vi "Joystickdrivemotor.vi"(6 "Max Output":dbl=1.0, 7 "Square Inputs":bool=TRUE, 8 "right y":dbl, 9 "Y axis value":dbl, 10 "X axis value":dbl) -> (0 "Boolean 2":bool, 1 "Right Motor Value":dbl, 2 "Left Motor Value":dbl)   [LabVIEW 2015]
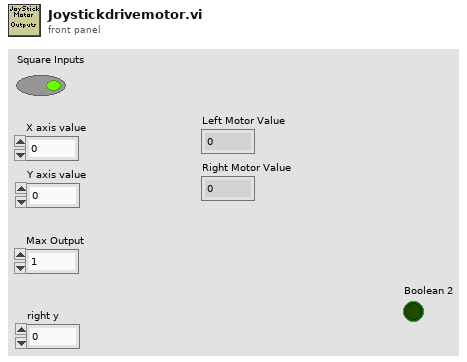
[diagram p1: front panel]
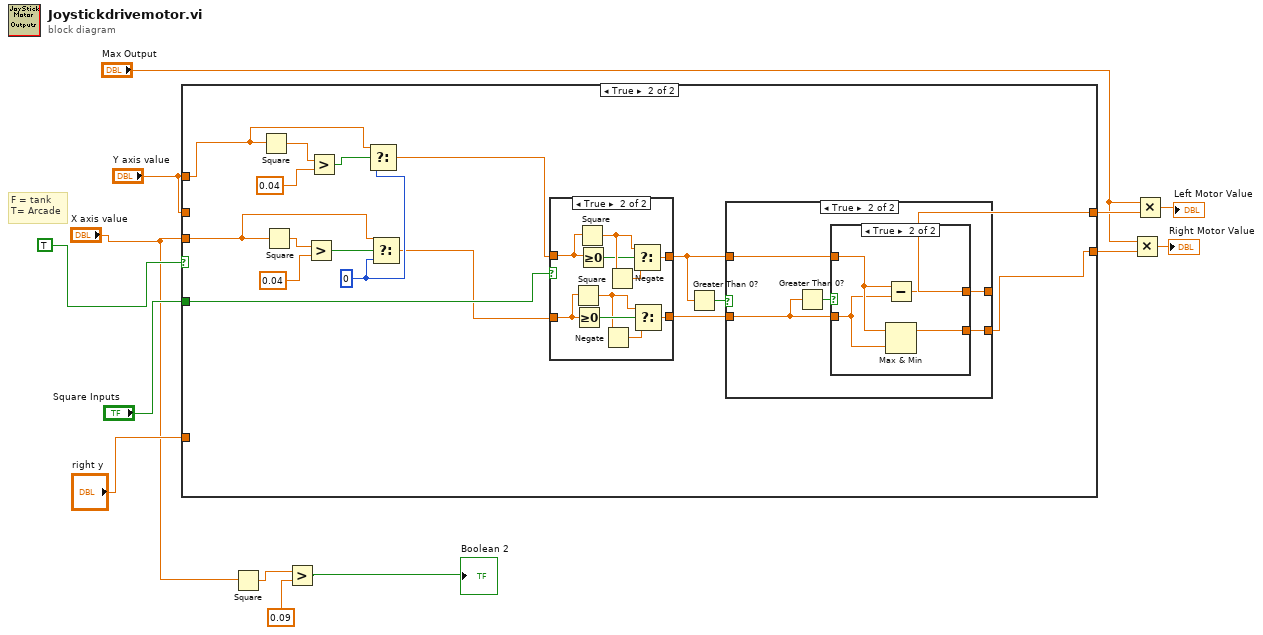
[diagram p0: block diagram]
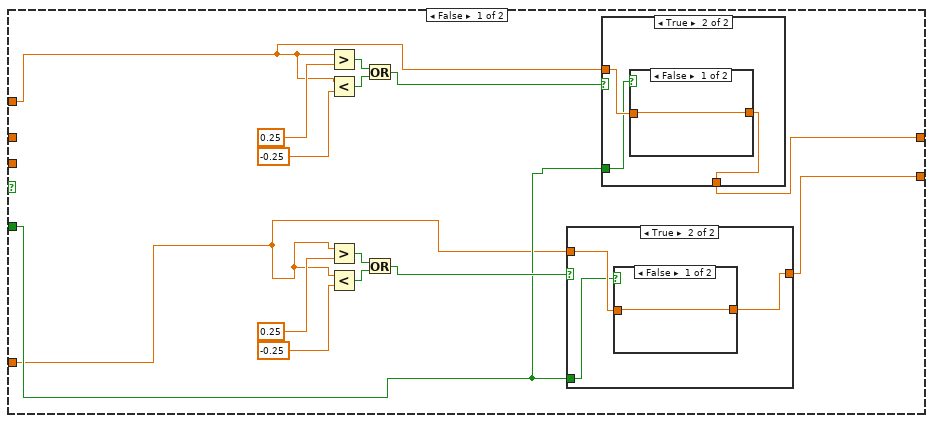
[diagram p2: hidden frame]
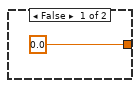
[diagram p3: hidden frame]
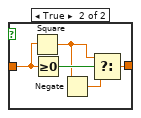
[diagram p4: hidden frame]
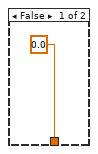
[diagram p5: hidden frame]
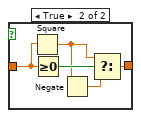
[diagram p6: hidden frame]
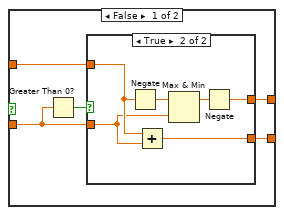
[diagram p7: hidden frame]
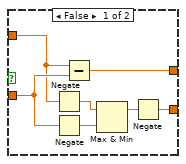
[diagram p8: hidden frame]
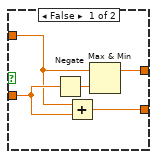
[diagram p9: hidden frame]
diagram:
  # "F = tank\nT= Arcade"
  n1 = case shown="True" TRUE {
    tunnel: [w15 w62] -> w13
    tunnel: "Y axis value" -> [w17 w57]
    tunnel: "X axis value" -> [_ w58]
    tunnel: [w14 w49] -> w12
    tunnel: "Square Inputs" -> [w18 w61]
    tunnel: "Y axis value" -> [_ _]
    tunnel: "right y" -> [w16 _]
    frame False {
      n2 = Greater?(x=w17, y=0.25) -> (0:w26:bool)
      n3 = Less?(x=w17, y=-0.25) -> (x < y?=w25:bool)
      n4 = Greater?(x=w16, y=0.25) -> (0:w21:bool)
      n5 = Less?(x=w16, y=-0.25) -> (x < y?=w20:bool)
      n6 = Or(x=w26, y=w25) -> (x .or. y?=w24:bool)
      n7 = Or(x=w21, y=w20) -> (x .or. y?=w19:bool)
      n8 = case shown="True" w19 {
        tunnel: [0.0 w32] -> w14
        tunnel: w16 -> [_ w31]
        tunnel: w18 -> [_ w30]
        frame False {
        }
        frame True {
          n9 = case shown="False" w30 {
            tunnel: [w33 w38] -> w32
            tunnel: w31 -> [w33 w37]
            frame False {
            }
            frame True {
              n10 = Square(x=w37) -> (x^2=w35:dbl)
              n11 = Greater Or Equal To 0?(x=w37) -> (x >= 0?=w36:bool)
              n12 = Negate(x=w35) -> (-x=w34:dbl)
              n13 = Select(t=w35, s=w36, f=w34) -> (s? t:f=w38:dbl)
            }
          }
        }
      }
      n14 = case shown="True" w24 {
        tunnel: [0.0 w42] -> w15
        tunnel: w17 -> [_ w41]
        tunnel: w18 -> [_ w40]
        frame False {
        }
        frame True {
          n15 = case shown="False" w40 {
            tunnel: [w43 w48] -> w42
            tunnel: w41 -> [w43 w47]
            frame False {
            }
            frame True {
              n16 = Square(x=w47) -> (x^2=w45:dbl)
              n17 = Greater Or Equal To 0?(x=w47) -> (x >= 0?=w46:bool)
              n18 = Negate(x=w45) -> (-x=w44:dbl)
              n19 = Select(t=w45, s=w46, f=w44) -> (s? t:f=w48:dbl)
            }
          }
        }
      }
    }
    frame True {
      w60 = 0
      n20 = Square(x=w57) -> (x^2=w53:dbl)
      n21 = Square(x=w58) -> (x^2=w55:dbl)
      n22 = Greater?(x=w55, y=0.04) -> (0:w50:bool)
      n23 = Greater?(x=w53, y=0.04) -> (0:w51:bool)
      n24 = Select(t=w57, s=w51, f=w60) -> (s? t:f=w59:dbl)
      n25 = Select(t=w58, s=w50, f=w60) -> (s? t:f=w56:dbl)
      n26 = case shown="True" w61 {
        tunnel: [w98 w109] -> w63
        tunnel: [w99 w108] -> w64
        tunnel: w56 -> [w98 w107]
        tunnel: w59 -> [w99 w106]
        frame False {
        }
        frame True {
          n27 = Square(x=w107) -> (x^2=w104:dbl)
          n28 = Greater Or Equal To 0?(x=w107) -> (x >= 0?=w105:bool)
          n29 = Square(x=w106) -> (x^2=w101:dbl)
          n30 = Greater Or Equal To 0?(x=w106) -> (x >= 0?=w100:bool)
          n31 = Negate(x=w104) -> (-x=w103:dbl)
          n32 = Negate(x=w101) -> (-x=w102:dbl)
          n33 = Select(t=w101, s=w100, f=w102) -> (s? t:f=w108:dbl)
          n34 = Select(t=w104, s=w105, f=w103) -> (s? t:f=w109:dbl)
        }
      }
      n35 = Greater Than 0?(x=w64) -> (x > 0?=w65:bool)
      n36 = case shown="True" w65 {
        tunnel: w63 -> [w69 w87]
        tunnel: w64 -> [w68 w86]
        tunnel: [w67 w85] -> w62
        tunnel: [w66 w84] -> w49
        frame False {
          n37 = Greater Than 0?(x=w69) -> (x > 0?=w70:bool)
          n38 = case shown="True" w70 {
            tunnel: w69 -> [w77 w79]
            tunnel: w68 -> [w75 w80]
            tunnel: [w71 w81] -> w67
            tunnel: [w72 w78] -> w66
            frame False {
              n39 = Negate(x=w75) -> (-x=w76:dbl)
              n40 = Negate(x=w77) -> (-x=w74:dbl)
              n41 = Subtract(x=w75, y=w77) -> (x-y=w71:dbl)
              n42 = Max & Min(x=w76, y=w74) -> (max(x,y)=w73:dbl)  [unwired: 1 out]
              n43 = Negate(x=w73) -> (-x=w72:dbl)
            }
            frame True {
              n44 = Negate(x=w80) -> (-x=w83:dbl)
              n45 = Add(x=w80, y=w79) -> (x+y=w78:dbl)
              n46 = Max & Min(x=w83, y=w79) -> (max(x,y)=w82:dbl)  [unwired: 1 out]
              n47 = Negate(x=w82) -> (-x=w81:dbl)
            }
          }
        }
        frame True {
          n48 = Greater Than 0?(x=w87) -> (x > 0?=w88:bool)
          n49 = case shown="True" w88 {
            tunnel: w87 -> [w93 w95]
            tunnel: w86 -> [w90 w96]
            tunnel: [w91 w94] -> w85
            tunnel: [w89 w97] -> w84
            frame False {
              n50 = Negate(x=w93) -> (-x=w92:dbl)
              n51 = Add(x=w90, y=w93) -> (x+y=w89:dbl)
              n52 = Max & Min(x=w90, y=w92) -> (max(x,y)=w91:dbl)  [unwired: 1 out]
            }
            frame True {
              n53 = Subtract(x=w96, y=w95) -> (x-y=w94:dbl)
              n54 = Max & Min(x=w96, y=w95) -> (max(x,y)=w97:dbl)  [unwired: 1 out]
            }
          }
        }
      }
    }
  }
  n55 = Square(x="X axis value") -> (x^2=w2:dbl)
  n56 = Greater?(x=w2, y=0.09) -> (0:→"Boolean 2":bool)
  n57 = Multiply(x="Max Output", y=w12) -> (x*y=→"Right Motor Value":dbl)
  n58 = Multiply(x="Max Output", y=w13) -> (x*y=→"Left Motor Value":dbl)
